vi "MicroPulse - Data Transmit.vi"(8 "error in (no error)":errorcluster, 10 "data":string, 11 "TCP config":T1={"Connection ID"=refnum, "IP address"="10.1.1.2", "host port"=1067, "OC timeout"=-1, "Read timeout"=0, "Write timeout"=0} {"Write timeout" format="%dms"; "Read timeout" format="%dms"; "OC timeout" format="%dms"}) -> (0 "error out":errorcluster, 2 "status  string":string, 3 "TCP config out":T1={"Connection ID"=refnum, "IP address"="10.1.1.2", "host port"=1067, "OC timeout"=-1, "Read timeout"=0, "Write timeout"=0} {"Write timeout" format="%dms"; "Read timeout" format="%dms"; "OC timeout" format="%dms"})   [LabVIEW 2026, in "MicroPulse_Driver.lvlib"]
doc: "Transmit commands to MicroPulse instrument.\nDoes nothing if <b>data</b> is empty."
uses:
  MicroPulse_Driver.lvlib
  Public/Data/Datatypes/TCP config.ctl
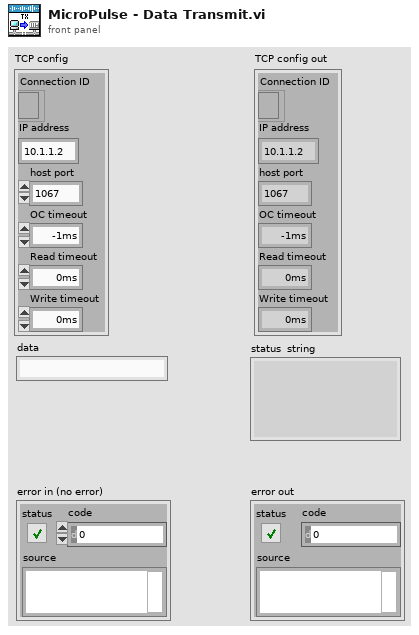
[diagram p1: front panel]
types:
  T1 = typedef "MicroPulse_Driver.lvlib/TCP config.ctl" = cluster{"Connection ID":refnum<k5>, "IP address":string, "host port":u16, "OC timeout":i32, "Read timeout":i32, "Write timeout":i32}
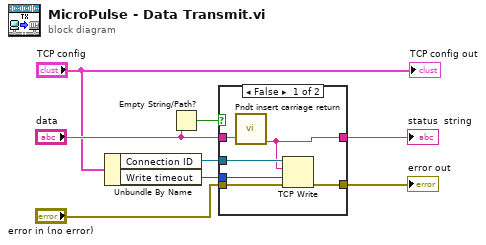
[diagram p0: block diagram]
diagram:
  n1 = Unbundle By Name("TCP config") -> ("Connection ID"=w3:refnum<k5>, "Write timeout"=w2:i32)
  n2 = Empty String/Path?(string/path="data") -> (empty?=w4:bool)
  n3 = case shown="False" w4 {
    tunnel: [w10 w15] -> w8
    tunnel: "data" -> [w14 w15]
    tunnel: [w13 w16] -> w7
    tunnel: "error in (no error)" -> [w12 w16]
    tunnel: w3 -> [w11 _]
    tunnel: w2 -> [w9 _]
    frame False {
      n4 = call "Pndt insert carriage return.vi"("transmit script"=w14) -> ("cmd script"=w10:string)  [unwired: 3 in, 1 out]
      n5 = TCP Write(connection ID=w11, data in=w10, error in (no error)=w12, 9:w9) -> (error out=w13:errorcluster)  [unwired: 2 out]
    }
    frame True {
    }
  }
  "status  string" <- w8
  "error out" <- w7
  "TCP config out" <- "TCP config"
